vi "Acctual_Step.vi"() -> ()   [LabVIEW 2017]
panel:
  out "acctualstep":dbl
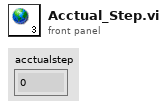
[diagram p1: front panel]
diagram:
